vi "GetImageInfo.vi"(8 "error in (no error)":errorcluster) -> (0 "error out":errorcluster, 1 "Y Resolution":i32, 2 "X Resolution":i32, 3 "Image Type":T1 items=["Grayscale (U8)", "Grayscale (I16)", "Grayscale (SGL)", "Complex (CSG)", "RGB (U32)", "HSL (U32)", "RGB (U64)", "Grayscale (U16)"], 4 "Return":i32)   [LabVIEW 2015]
uses:
  [Global] Image.vi
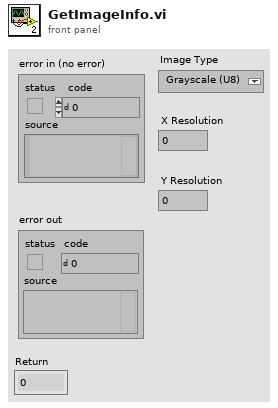
[diagram p1: front panel]
types:
  T1 = typedef "Image Type" = u32
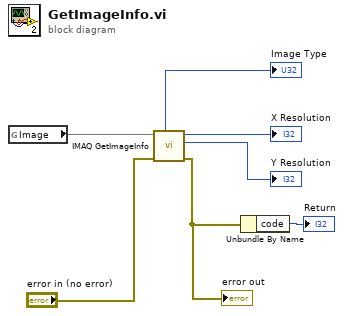
[diagram p0: block diagram]
diagram:
  n1 = global read "[Global] Image.vi" "Image"() -> (w7)
  n2 = call "IMAQ GetImageInfo"("error in (no error)"="error in (no error)", "Image"=w7) -> ("error out"=w3:errorcluster, "Y Resolution"=→"Y Resolution":i32, "X Resolution"=→"X Resolution":i32, "Image Type"=→"Image Type":T1)  [unwired: 2 in, 4 out]
  "error out" <- w3
  n3 = Unbundle By Name(w3) -> ("code"=→"Return":i32)
